vi "piano UI 2.vi"() -> ()   [LabVIEW 2020]
uses:
  midi/midi.lvclass
  midi-file/midi-file.lvclass
  midi-ui/midi-ui.lvclass
  midi/midi.lvclass/midi.ctl
  midi-ui/midi-ui.lvclass/midi-ui.ctl
  <vilib>/addons/_JKI Toolkits/State Machine/_JKI_lib_State_Machine.llb/Select State(s)_err__jki_lib_state_machine.vi
panel:
  in  "Pause":bool
  in  "Stop":bool
  out "Connected?":bool
  in  "Play":bool
  in  "MIDI Out Channel":u32
  in  "Connect MIDI OUT":bool
  in  "Note Length (-1)":dbl=50.0 format="%#_13g"
  in  "Position":enum16{"Top", "Left", "Botom", "Right"}(ring)=enum."Left"
  in  "Load File":bool
  in  "Exit":bool
  out "picture":picture
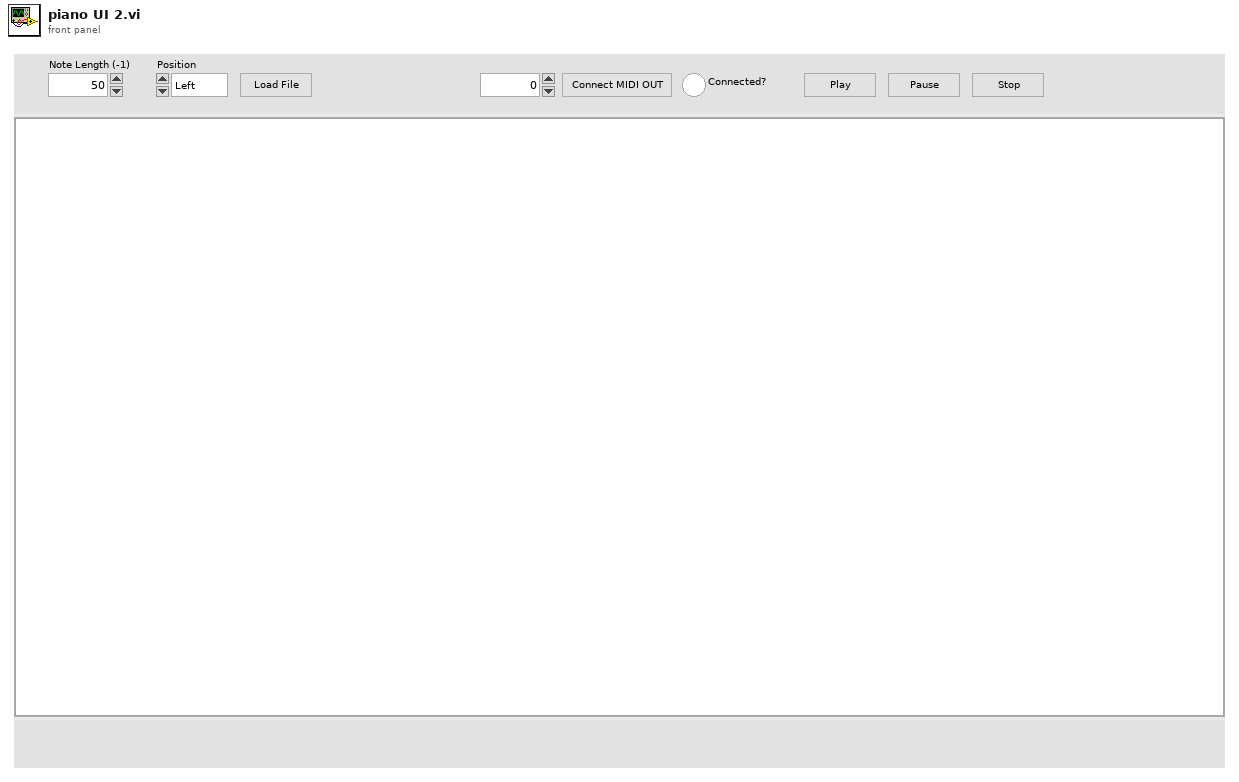
[diagram p1: front panel]
types:
  T1 = enum32{"Invalid", "Standard", "Closed", "Hidden", "Minimized", "Maximized"}
  T2 = enum32{"invalid app kind", "Development System", "Run Time System", "Student Edition", "Embedded LabVIEW", "Evaluation", "Custom"}
  T3 = cluster{"Core":cluster{"Current VI Reference":refnum<vi>, "Close Panel on Exit?":bool}, "MIDI UI obj":refnum<class "midi-ui.lvclass">, "file events":cluster{"Time Delay":u32, "MIDI Messages":u16, "Note Value":enum8{"C-2", "C#-2", "D-2", "D#-2", "E-2", "F-2", "F#-2", "G-2", "G#-2", "A-2", "A#-2", "B-2", "C-1", "C#-1", "D-1", "D#-1", "E-1", "F-1", "F#-1", "G-1", "G#-1", "A-1", "A#-1", "B-1", "C0", "C#0", "D0", "D#0", "E0", "F0", "F#0", "G0", "G#0", "A0", "A#0", "B0", "C1", "C#1", "D1", "D#1", "E1", "F1", "F#1", "G1", "G#1", "A1", "A#1", "B1", "C2", "C#2", "D2", "D#2", "E2", "F2", "F#2", "G2", "G#2", "A2", "A#2", "B2", "C3", "C#3", "D3", "D#3", "E3", "F3", "F#3", "G3", "G#3", "A3", "A#3", "B3", "C4", "C#4", "D4", "D#4", "E4", "F4", "F#4", "G4", "G#4", "A4", "A#4", "B4", "C5", "C#5", "D5", "D#5", "E5", "F5", "F#5", "G5", "G#5", "A5", "A#5", "B5", "C6", "C#6", "D6", "D#6", "E6", "F6", "F#6", "G6", "G#6", "A6", "A#6", "B6", "C7", "C#7", "D7", "D#7", "E7", "F7", "F#7", "G7", "G#7", "A7", "A#7", "B7", "C8", "C#8", "D8", "D#8", "E8", "F8", "F#8", "G"}, "Volume":u8, "uid":i32}[], "file meta events":cluster{"Delta Tiime":u32, "MIDI Meta Events":u16, "String Data":string, "Numeric Data":i32[]}[], "MIDI FILE obj":refnum<class "midi-file.lvclass">, "midi obj":refnum<class "midi.lvclass">, "midi connected?":bool}
  T4 = cluster{"Time Delay":u32, "MIDI Messages":u16, "Note Value":enum8{"C-2", "C#-2", "D-2", "D#-2", "E-2", "F-2", "F#-2", "G-2", "G#-2", "A-2", "A#-2", "B-2", "C-1", "C#-1", "D-1", "D#-1", "E-1", "F-1", "F#-1", "G-1", "G#-1", "A-1", "A#-1", "B-1", "C0", "C#0", "D0", "D#0", "E0", "F0", "F#0", "G0", "G#0", "A0", "A#0", "B0", "C1", "C#1", "D1", "D#1", "E1", "F1", "F#1", "G1", "G#1", "A1", "A#1", "B1", "C2", "C#2", "D2", "D#2", "E2", "F2", "F#2", "G2", "G#2", "A2", "A#2", "B2", "C3", "C#3", "D3", "D#3", "E3", "F3", "F#3", "G3", "G#3", "A3", "A#3", "B3", "C4", "C#4", "D4", "D#4", "E4", "F4", "F#4", "G4", "G#4", "A4", "A#4", "B4", "C5", "C#5", "D5", "D#5", "E5", "F5", "F#5", "G5", "G#5", "A5", "A#5", "B5", "C6", "C#6", "D6", "D#6", "E6", "F6", "F#6", "G6", "G#6", "A6", "A#6", "B6", "C7", "C#7", "D7", "D#7", "E7", "F7", "F#7", "G7", "G#7", "A7", "A#7", "B7", "C8", "C#8", "D8", "D#8", "E8", "F8", "F#8", "G"}, "Volume":u8, "uid":i32}[]
  T5 = cluster{"Delta Tiime":u32, "MIDI Meta Events":u16, "String Data":string, "Numeric Data":i32[]}[]
  T6 = cluster{"Current VI Reference":refnum<vi>, "Close Panel on Exit?":bool}
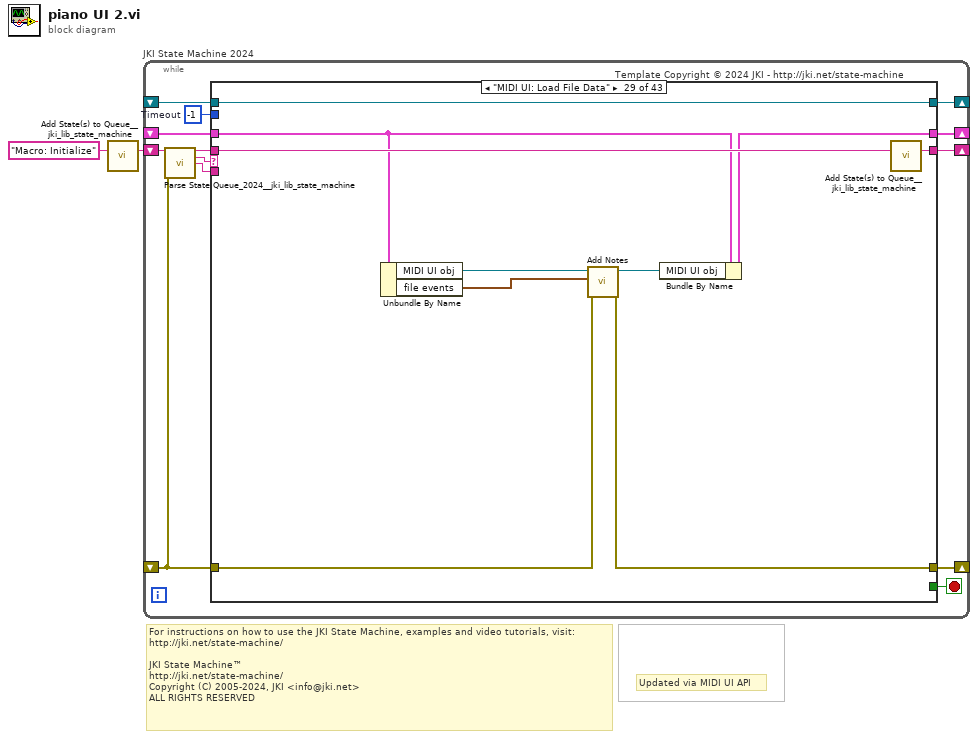
[diagram p0: block diagram]
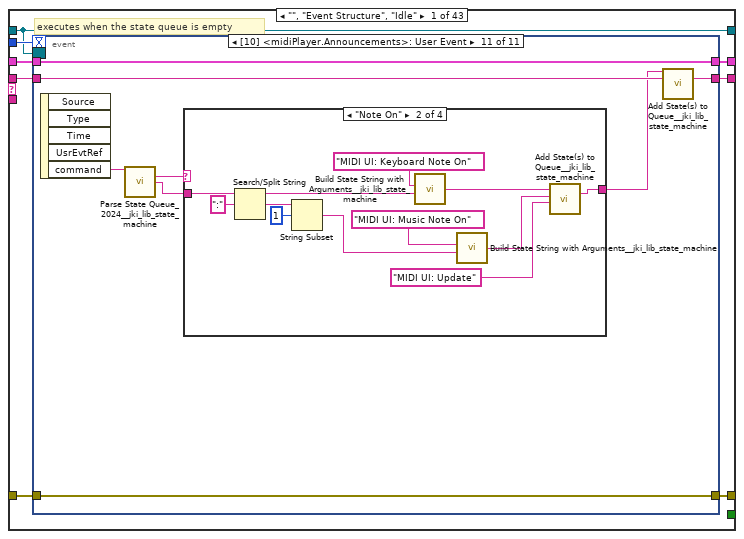
[diagram p2: hidden frame]
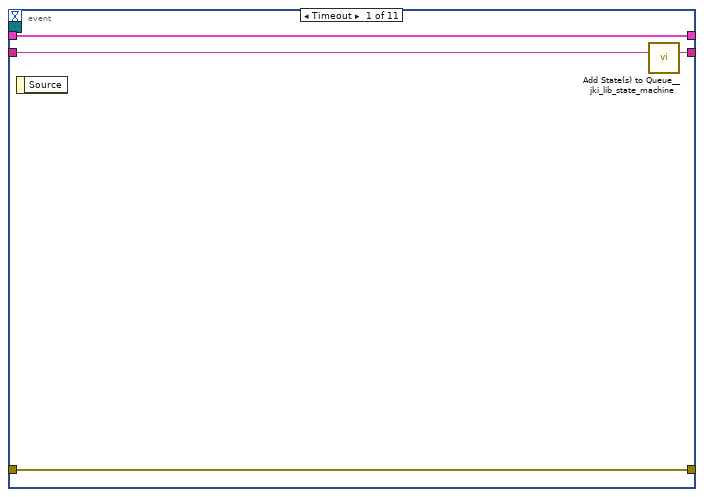
[diagram p3: hidden frame]
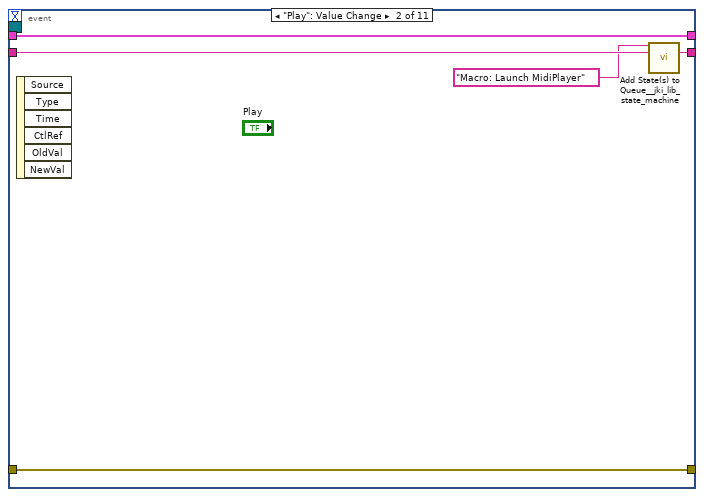
[diagram p4: hidden frame]
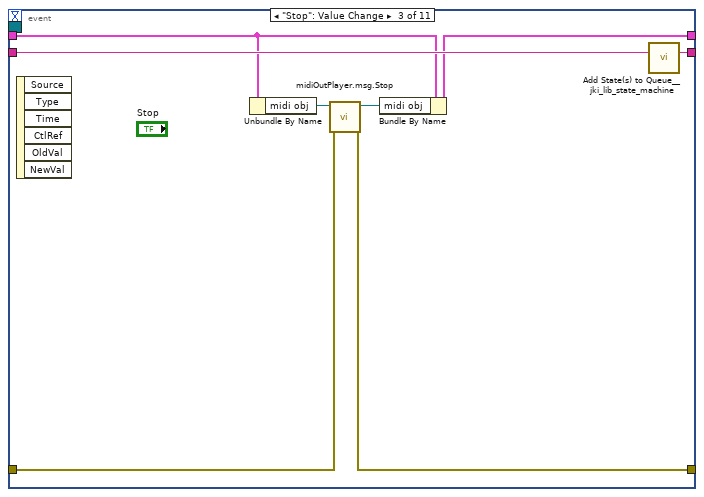
[diagram p5: hidden frame]
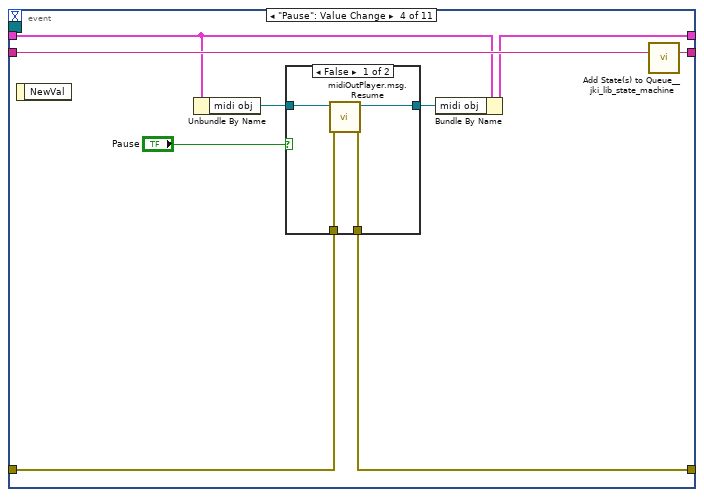
[diagram p6: hidden frame]
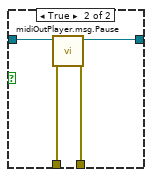
[diagram p7: hidden frame]
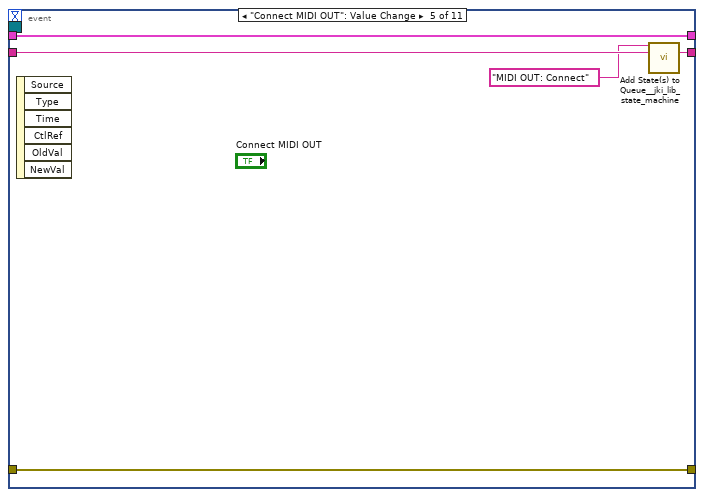
[diagram p8: hidden frame]
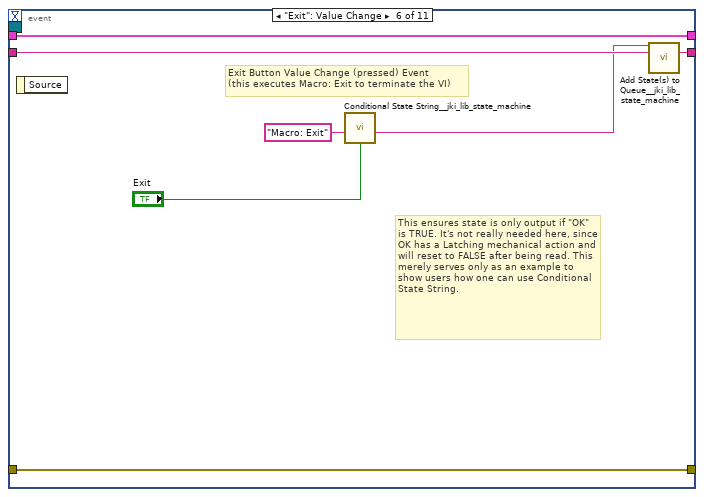
[diagram p9: hidden frame]
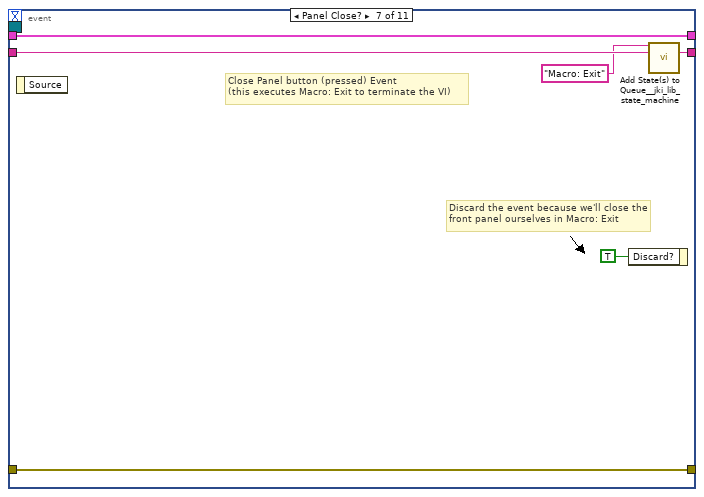
[diagram p10: hidden frame]
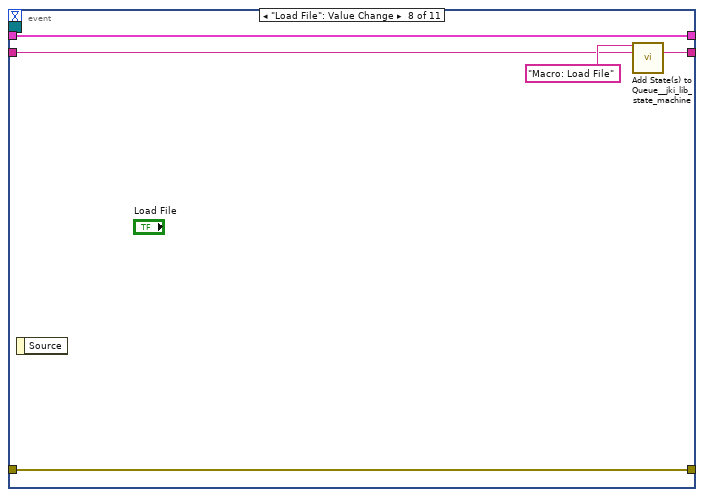
[diagram p11: hidden frame]
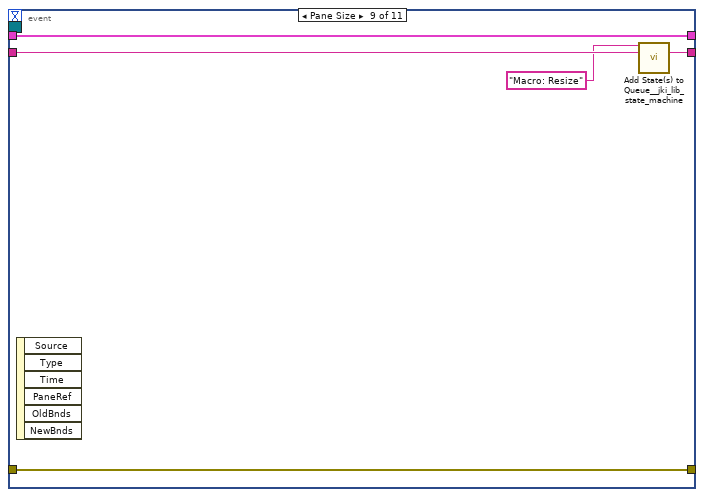
[diagram p12: hidden frame]
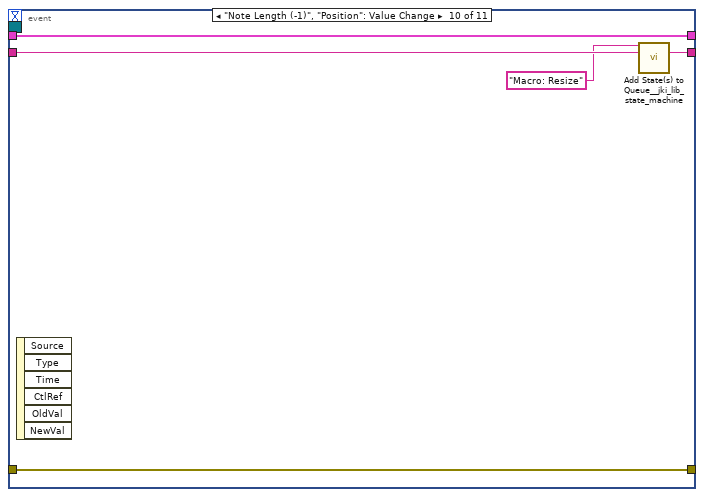
[diagram p13: hidden frame]
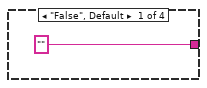
[diagram p14: hidden frame]
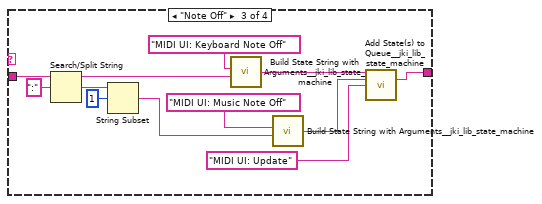
[diagram p15: hidden frame]
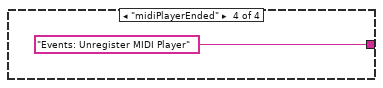
[diagram p16: hidden frame]
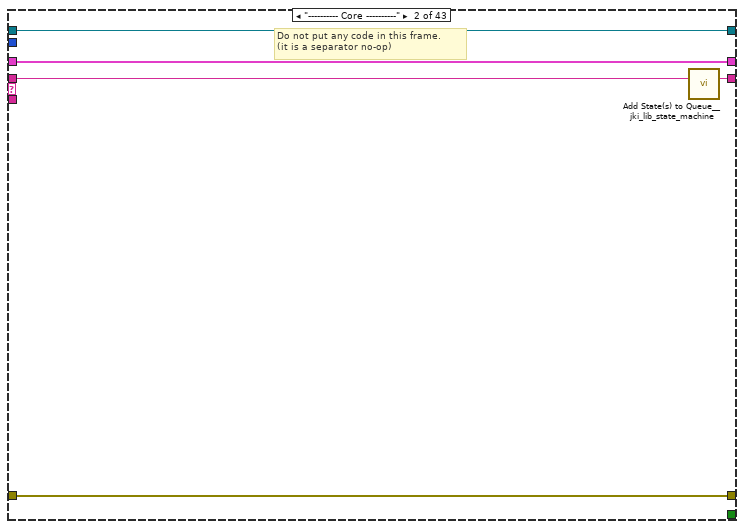
[diagram p17: hidden frame]
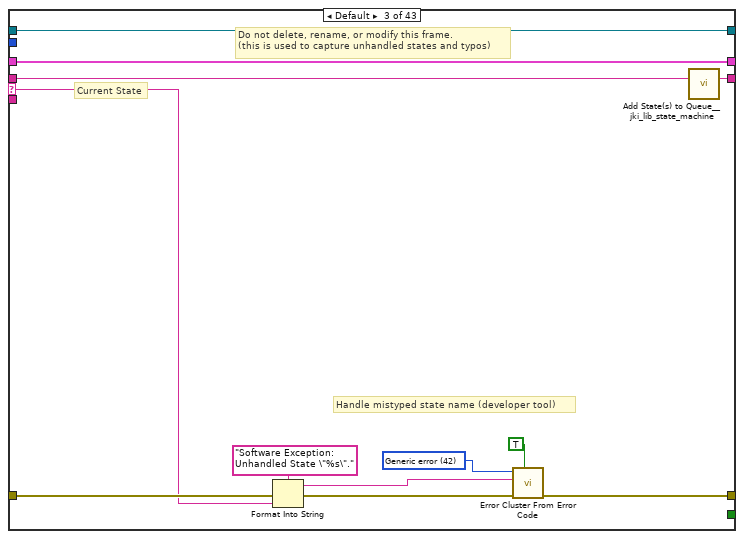
[diagram p18: hidden frame]
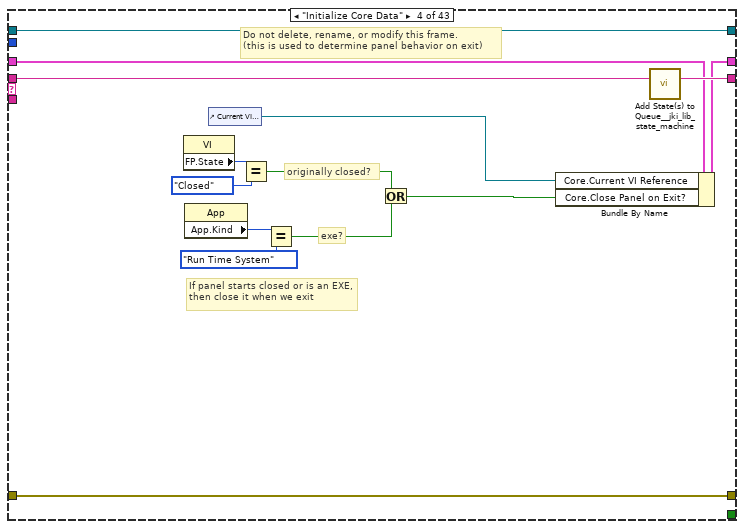
[diagram p19: hidden frame]
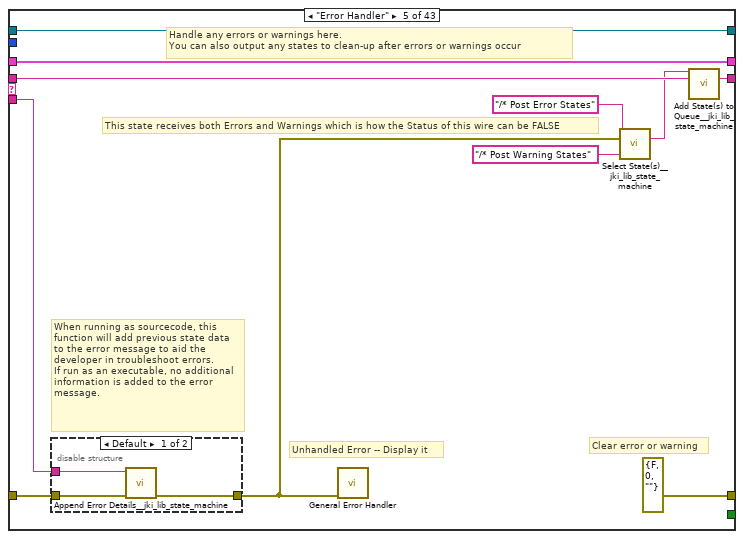
[diagram p20: hidden frame]
diagram:
  # "Updated via MIDI UI API"
  # "For instructions on how to use the JKI State Machine, examples and video tutorials, visit:\nhttp://jki.net/state-machine/\n\nJKI State Machine™\nhttp://jki.net/state-machine/\nCopyright (C) 2005-2024, JKI <info@jki.net>\nALL RIGHTS RESERVED"
  n1 = call <vilib>:"Add State(s) to Queue__jki_lib_state_machine.vi"("State(s) in (\"\")"="Macro: Initialize") -> ("States Out"=w2:string)  [unwired: 14 in]
  n2 = while "JKI State Machine 2024" {
    shift-right: [w10] -> _
    shift-left: _ -> [w9]
    shift-right: [w13] -> _
    shift-left: _ -> [w7]
    shift-right: [w12] -> _
    shift-left: w2 -> [w14]
    shift-right: [w4] -> _
    shift-left: _ -> [w3]
    stop <- w11 stop-if-true
    w8 = -1  # Timeout
    # "Template Copyright © 2024 JKI - http://jki.net/state-machine"
    n3 = call <vilib>:"Parse State Queue_2024__jki_lib_state_machine.vi"("State Queue"=w14, "Error In (no error)"=w7) -> ("Remaining States"=w15:string, "Current State"=w5:string, "Arguments"=w6:string)  [unwired: 11 in]
    n4 = case shown="\"MIDI UI: Load File Data\"" w5 {
      selector: w5 -> [_ _ w131 _ _ _ _ _ _ _ _ _ _ _ _ _ _ _ _ _ _ _ _ _ _ _ _ _ _ _ _ _ _ _ _ _ _ _ _ _ _ _ _]
      tunnel: w15 -> [w23 w129 w135 w155 w166 w176 w181 w198 w205 w210 w217 w226 w234 w240 w245 w251 w256 w263 w275 w345 w351 w357 w363 w369 w382 w387 w394 w408 w418 w430 w440 w450 w460 w470 w473 w482 w493 w500 w505 w516 w526 w536 w545]
      tunnel: w6 -> [_ _ _ _ w161 _ _ _ _ _ _ _ _ _ _ _ _ w258 w269 _ _ _ _ _ _ _ _ _ _ _ w433 w443 w453 w463 _ _ _ _ _ _ _ _ _]
      tunnel: w9 -> [w21 w126 w133 w148 w163 w174 w178 _ w200 w207 w215 w221 w232 w238 w242 w249 w254 w261 w271 w342 w348 w354 w360 w366 w380 w384 w391 w404 w411 w422 w438 w448 w458 w468 w475 w480 w489 w499 w504 w511 w522 w530 w541]
      tunnel: [w20 w127 w137 w152 errorcluster {"status"=FALSE, "code"=0, "source"=""} ("error out") w173 w179 w190 w201 w208 w214 w224 w231 w235 w243 w248 w253 w259 w272 w343 w349 w355 w361 w367 w377 w385 w388 w401 w410 w424 w431 w441 w451 w461 w472 w478 w486 w496 w503 w508 w520 w531 w539] -> w13
      tunnel: w7 -> [w17 w127 w136 w152 w162 w173 w179 w193 w202 w208 w213 w223 w230 w236 w243 w248 w253 w260 w273 w343 w349 w355 w361 w367 w377 w385 w388 w396 w414 w425 w432 w442 w452 w462 w472 w481 w487 w497 w503 w514 w521 w532 w540]
      tunnel: [w22 w128 w134 w154 w165 w175 w180 w197 w204 w209 w216 w225 w233 w239 w244 w250 w255 w262 w274 w344 w350 w356 w362 w368 w381 w386 w393 w407 w417 w429 w439 w449 w459 w469 w474 w483 w494 w501 w506 w517 w527 w537 w546] -> w12
      tunnel: [_ _ _ _ _ TRUE _ _ _ _ _ _ _ _ _ _ _ _ _ _ _ _ _ _ _ _ _ _ _ _ _ _ _ _ _ _ _ _ _ _ _ _ _] -> w11
      tunnel: [w19 w126 w133 w153 w163 w174 w178 w196 w200 w207 w215 w221 w232 w238 w242 w249 w254 w261 w271 w342 w348 w354 w360 w366 w380 w384 w391 w403 w412 w421 w437 w447 w457 w467 w475 w479 w492 w499 w504 w512 w525 w529 w538] -> w10
      tunnel: w8 -> [w18 _ _ _ _ _ _ _ _ _ _ _ _ _ _ _ _ _ _ _ _ _ _ _ _ _ _ _ _ _ _ _ _ _ _ _ _ _ _ _ _ _ _]
      tunnel: [w16 w125 w130 w142 w156 w171 w177 w184 w199 w206 w211 w219 w227 w237 w241 w247 w252 w257 w268 w341 w347 w352 w358 w364 w374 w383 w392 w395 w409 w419 w436 w446 w456 w466 w471 w476 w484 w495 w502 w509 w519 w535 w544] -> w4
      tunnel: w3 -> [w16 w125 w130 w142 w156 w171 w177 w184 w199 w206 w212 w218 w229 w237 w241 w247 w252 w257 w268 w341 w347 w352 w358 w364 w374 w383 w392 w395 w409 w419 w436 w446 w456 w466 w471 w476 w484 w495 w502 w509 w519 w535 w544]
      frame "", "Event Structure", "Idle" {
        # "executes when the state queue is empty"
        n5 = event shown="[10] <midiPlayer.Announcements>: User Event" {
          selector: w16 -> [_ _ _ _ _ _ _ _ _ _ _]
          dyn-events: _ -> [_ _ _ _ _ _ _ _ _ _ _]
          timeout: w18 -> [_ _ _ _ _ _ _ _ _ _ _]
          tunnel: w23 -> [w27 w32 w40 w49 w62 w69 w75 w79 w83 w88 w96]
          tunnel: [w26 w31 w39 w48 w61 w68 w74 w78 w84 w89 w97] -> w22
          tunnel: w21 -> [w24 w29 w37 w46 w59 w66 w72 w77 w85 w90 w91]
          tunnel: [w25 w30 w33 w42 w60 w67 w73 w76 w82 w87 w98] -> w20
          tunnel: w17 -> [w25 w30 w34 w43 w60 w67 w73 w76 w82 w87 w98]
          tunnel: [w24 w29 w36 w45 w59 w66 w72 w77 w85 w90 w91] -> w19
          event Timeout {
            n6 = event-data() -> ()  [unwired: 1 in, 1 out]
            n7 = call <vilib>:"Add State(s) to Queue__jki_lib_state_machine.vi"("State(s) in (\"\")"=w27) -> ("States Out"=w26:string)  [unwired: 14 in]
          }
          event "Play": Value Change {
            n8 = event-data() -> ()  [unwired: 1 in, 6 out]
            n9 = call <vilib>:"Add State(s) to Queue__jki_lib_state_machine.vi"("State(s) in Front (\"\")"="Macro: Launch MidiPlayer" ("State(s) in Front (\"\")"), "State(s) in (\"\")"=w32) -> ("States Out"=w31:string)  [unwired: 13 in]
          }
          event "Stop": Value Change {
            n10 = event-data() -> ()  [unwired: 1 in, 6 out]
            n11 = Unbundle By Name(w37) -> ("midi obj"=w38:refnum<class "midi.lvclass">)
            n12 = call "midiOutPlayer.msg.Stop.vi"("error in (no error)"=w34, "midi in"=w38) -> ("error out"=w33:errorcluster, "midi out"=w35:refnum<class "midi.lvclass">)  [unwired: 8 in]
            n13 = Bundle By Name(cluster=w37, "midi obj"=w35) -> (w36:T3)
            n14 = call <vilib>:"Add State(s) to Queue__jki_lib_state_machine.vi"("State(s) in (\"\")"=w40) -> ("States Out"=w39:string)  [unwired: 14 in]
          }
          event "Pause": Value Change {
            n15 = event-data() -> ()  [unwired: 1 in, 1 out]
            n16 = Unbundle By Name(w46) -> ("midi obj"=w47:refnum<class "midi.lvclass">)
            n17 = case shown="False" "Pause" {
              tunnel: w47 -> [w53 w57]
              tunnel: [w51 w56] -> w44
              tunnel: w43 -> [w52 w55]
              tunnel: [w50 w54] -> w42
              frame False {
                n18 = call "midiOutPlayer.msg.Resume.vi"("error in (no error)"=w52, "midi in"=w53) -> ("error out"=w50:errorcluster, "midi out"=w51:refnum<class "midi.lvclass">)  [unwired: 8 in]
              }
              frame True {
                n19 = call "midiOutPlayer.msg.Pause.vi"("error in (no error)"=w55, "midi in"=w57) -> ("error out"=w54:errorcluster, "midi out"=w56:refnum<class "midi.lvclass">)  [unwired: 8 in]
              }
            }
            n20 = Bundle By Name(cluster=w46, "midi obj"=w44) -> (w45:T3)
            n21 = call <vilib>:"Add State(s) to Queue__jki_lib_state_machine.vi"("State(s) in (\"\")"=w49) -> ("States Out"=w48:string)  [unwired: 14 in]
          }
          event "Connect MIDI OUT": Value Change {
            n22 = event-data() -> ()  [unwired: 1 in, 6 out]
            n23 = call <vilib>:"Add State(s) to Queue__jki_lib_state_machine.vi"("State(s) in Front (\"\")"="MIDI OUT: Connect" ("State(s) in Front (\"\")"), "State(s) in (\"\")"=w62) -> ("States Out"=w61:string)  [unwired: 13 in]
          }
          event "Exit": Value Change {
            # "This ensures state is only output if \"OK\" is TRUE. It's not really needed here, since OK has a Latching mechanical action and will reset to FALSE after being read. This merely serves only as an example to show users how one can use Conditional State String."
            # "Exit Button Value Change (pressed) Event\n(this executes Macro: Exit to terminate the VI)"
            n24 = event-data() -> ()  [unwired: 1 in, 1 out]
            n25 = call <vilib>:"Conditional State String__jki_lib_state_machine.vi"("Do State(s)?"="Exit", "State"="Macro: Exit") -> ("State Out"=w63:string)  [unwired: 7 in]
            n26 = call <vilib>:"Add State(s) to Queue__jki_lib_state_machine.vi"("State(s) in Front (\"\")"=w63, "State(s) in (\"\")"=w69) -> ("States Out"=w68:string)  [unwired: 13 in]
          }
          event Panel Close? {
            # "Discard the event because we'll close the front panel ourselves in Macro: Exit"
            # "Close Panel button (pressed) Event\n(this executes Macro: Exit to terminate the VI)"
            n27 = event-data() -> ()  [unwired: 1 in, 1 out]
            n28 = event-data("Discard?"=TRUE) -> ()  [unwired: 1 in, 1 out]
            n29 = call <vilib>:"Add State(s) to Queue__jki_lib_state_machine.vi"("State(s) in Front (\"\")"="Macro: Exit", "State(s) in (\"\")"=w75) -> ("States Out"=w74:string)  [unwired: 13 in]
          }
          event "Load File": Value Change {
            n30 = event-data() -> ()  [unwired: 1 in, 1 out]
            n31 = call <vilib>:"Add State(s) to Queue__jki_lib_state_machine.vi"("State(s) in Front (\"\")"="Macro: Load File", "State(s) in (\"\")"=w79) -> ("States Out"=w78:string)  [unwired: 13 in]
          }
          event Pane Size {
            n32 = event-data() -> ()  [unwired: 1 in, 6 out]
            n33 = call <vilib>:"Add State(s) to Queue__jki_lib_state_machine.vi"("State(s) in Front (\"\")"="Macro: Resize" ("State(s) in Front (\"\")"), "State(s) in (\"\")"=w83) -> ("States Out"=w84:string)  [unwired: 13 in]
          }
          event "Note Length (-1)", "Position": Value Change {
            n34 = event-data() -> ()  [unwired: 1 in, 6 out]
            n35 = call <vilib>:"Add State(s) to Queue__jki_lib_state_machine.vi"("State(s) in Front (\"\")"="Macro: Resize" ("State(s) in Front (\"\")"), "State(s) in (\"\")"=w88) -> ("States Out"=w89:string)  [unwired: 13 in]
          }
          event User Event {
            n36 = event-data() -> ("command"=w95:string)  [unwired: 1 in, 4 out]
            n37 = call <vilib>:"Parse State Queue_2024__jki_lib_state_machine.vi"("State Queue"=w95) -> ("Current State"=w94:string, "Arguments"=w92:string)  [unwired: 12 in, 1 out]
            n38 = case shown="\"Note On\"" w94 {
              tunnel: ["" ("State(s) in Front (\"\")") w101 w123 "Events: Unregister MIDI Player" ("State(s) in Front (\"\")")] -> w93
              tunnel: w92 -> [_ w100 w118 _]
              frame "False", Default {
              }
              frame "Note On" {
                n39 = Search/Split String(string=w100, search string/char (-)=":") -> (substring before match=w108:string, match + rest of string=w107:string)  [unwired: 1 in, 1 out]
                n40 = String Subset(string=w107, offset (0)=1) -> (substring=w103:string)  [unwired: 1 in]
                n41 = call <vilib>:"Build State String with Arguments__jki_lib_state_machine.vi"("Arguments (\"\")"=w108, "State"="MIDI UI: Keyboard Note On" ("State(s) in Front (\"\")")) -> ("State with Arguments"=w110:string)  [unwired: 4 in]
                n42 = call <vilib>:"Build State String with Arguments__jki_lib_state_machine.vi"("Arguments (\"\")"=w103, "State"="MIDI UI: Music Note On" ("State(s) in Front (\"\")")) -> ("State with Arguments"=w102:string)  [unwired: 4 in]
                n43 = call <vilib>:"Add State(s) to Queue__jki_lib_state_machine.vi"("State(s) in Front (\"\")"=w110, "State(s) in (\"\")"=w102, "State(s) at Back (\"\")"="MIDI UI: Update" ("State(s) in (\"\")")) -> ("States Out"=w101:string)  [unwired: 12 in]
              }
              frame "Note Off" {
                n44 = Search/Split String(string=w118, search string/char (-)=":") -> (substring before match=w119:string, match + rest of string=w117:string)  [unwired: 1 in, 1 out]
                n45 = String Subset(string=w117, offset (0)=1) -> (substring=w113:string)  [unwired: 1 in]
                n46 = call <vilib>:"Build State String with Arguments__jki_lib_state_machine.vi"("Arguments (\"\")"=w119, "State"="MIDI UI: Keyboard Note Off" ("State(s) in Front (\"\")")) -> ("State with Arguments"=w121:string)  [unwired: 4 in]
                n47 = call <vilib>:"Build State String with Arguments__jki_lib_state_machine.vi"("Arguments (\"\")"=w113, "State"="MIDI UI: Music Note Off" ("State(s) in Front (\"\")")) -> ("State with Arguments"=w112:string)  [unwired: 4 in]
                n48 = call <vilib>:"Add State(s) to Queue__jki_lib_state_machine.vi"("State(s) in Front (\"\")"=w121, "State(s) in (\"\")"=w112, "State(s) at Back (\"\")"="MIDI UI: Update" ("State(s) in (\"\")")) -> ("States Out"=w123:string)  [unwired: 12 in]
              }
              frame "midiPlayerEnded" {
              }
            }
            n49 = call <vilib>:"Add State(s) to Queue__jki_lib_state_machine.vi"("State(s) in Front (\"\")"=w93, "State(s) in (\"\")"=w96) -> ("States Out"=w97:string)  [unwired: 13 in]
          }
        }
      }
      frame "---------- Core ----------" {
        # "Do not put any code in this frame.\n(it is a separator no-op)"
        n50 = call <vilib>:"Add State(s) to Queue__jki_lib_state_machine.vi"("State(s) in (\"\")"=w129) -> ("States Out"=w128:string)  [unwired: 14 in]
      }
      frame Default {
        w140 = 42 items=["No error", "Argument error", "Memory is full", "Out of zone", "End of file", "File already open", "Generic file I/O error", "File not found", "File permission error", "Disk is full", "Duplicate path", "Too many files open", "System feature not enabled", "Resource file not found", "Cannot add resource", "Resource not found", "Image not found", "Image memory error", "Pen does not exist", "Config type invalid", "Config token not found", "Config parse error", "Config memory error", "Bad external code format", "Bad external code offset", "External code not present", "Null window", "Destroy window error", "Null menu", "Print aborted", "Bad print record", "Print driver error", "Windows error during printing", "Memory error during printing", "Print dialog error", "Generic print error", "Invalid device refnum", "Device not found", "Device parameter error", "Device unit error", "Cannot open device", "Device call aborted", "Generic error", "Cancelled by user", "Object ID too low", "Object ID too high", "Object not in heap", "Unknown heap", "Unknown object (invalid DefProc)", "Unknown object (DefProc not in table)", "Message out of range", "Invalid (null) method", "Unknown message", "Manager call not supported", "Bad address", "Network operation in progress", "Network operation timed out", "Connection is busy", "Network attribute not supported", "Network error", "Address in use", "System out of memory", "Connection aborted", "Connection refused", "Not connected", "Already connected", "Connection closed", "Initialization error (interapplication manager)", "Bad occurrence", "Wait on unbound occurrence handler", "Occurrence queue overflow", "Datalog type conflict", "Unused", "Unrecognized type (interapplication manager)", "Memory corrupt", "Failed to make temporary DLL", "Old CIN version", "Drag socket not found", "Failed to load drop-object", "Failed to register OLE object", "Failed to release OLE object", "Format specifier type mismatch", "Unknown format specifier", "Too few format specifiers", "Too many format specifiers", "Scan failed", "Newer CIN version", "Error converting to variant", "Runtime menu error", "Password tampered", "Variant attribute not found", "Incompatible variant data type", "Event data is not available", "Event Store is not present", "Occurrence is not found", "Event Queue is not created", "Event info is not available", "Refnum passed is NULL", "Error retrieving Class GUID", "Error retrieving CoClass GUID", "Error retrieving TypeLib GUID.", "Bad built application magic bytes.", "Specific driver is different from the specific driver associated with the Logical Name.", "There is no session opened to the class driver.", "Max Error", "MAX - Error with config objects", "MAX - Error loading configuration", "MAX - Group not supported"]
        # "Current State"
        # "Do not delete, rename, or modify this frame.\n(this is used to capture unhandled states and typos)"
        # "Handle mistyped state name (developer tool)"
        n51 = Format Into String(format string="Software Exception: Unhandled State \"%s\"." ("message"), error in=w136, w131) -> (resulting string=w139:string, error out=w138:errorcluster)  [unwired: 1 in]
        n52 = call <vilib>:"Error Cluster From Error Code.vi"("show call chain? (False)"=TRUE, "error in (no error)"=w138, "error message (\"\")"=w139, "error code (0)"=w140) -> ("error out"=w137:errorcluster)  [unwired: 5 in]
        n53 = call <vilib>:"Add State(s) to Queue__jki_lib_state_machine.vi"("State(s) in (\"\")"=w135) -> ("States Out"=w134:string)  [unwired: 14 in]
      }
      frame "Initialize Core Data" {
        # "Do not delete, rename, or modify this frame.\n(this is used to determine panel behavior on exit)"
        # "originally closed?"
        # "exe?"
        # "If panel starts closed or is an EXE, then close it when we exit"
        n54 = property class="VI"() -> ("FP.State"=w145:T1)  [unwired: 2 in, 2 out]
        n55 = property class="App"() -> ("App.Kind"=w151:T2)  [unwired: 2 in, 2 out]
        n56 = control-ref of="Current VI Reference"() -> (w146:refnum<vi>)
        n57 = Equal?(x=w145, y=T1."Closed" ("Front Panel Window:State")) -> (x = y?=w143:bool)
        n58 = Equal?(x=w151, y=T2."Run Time System" ("Application:Kind")) -> (x = y?=w149:bool)
        n59 = Or(x=w143, y=w149) -> (x .or. y?=w147:bool)
        n60 = Bundle By Name(cluster=w148, "Core.Current VI Reference"=w146, "Core.Close Panel on Exit?"=w147) -> (w153:T3)
        n61 = call <vilib>:"Add State(s) to Queue__jki_lib_state_machine.vi"("State(s) in (\"\")"=w155) -> ("States Out"=w154:string)  [unwired: 14 in]
      }
      frame "Error Handler" {
        # "When running as sourcecode, this function will add previous state data to the error message to aid the developer in troubleshoot errors.\nIf run as an executable, no additional information is added to the error message."
        # "This state receives both Errors and Warnings which is how the Status of this wire can be FALSE"
        # "Unhandled Error -- Display it"
        # "Handle any errors or warnings here.\nYou can also output any states to clean-up after errors or warnings occur"
        # "Clear error or warning"
        n62 = disable-structure shown="Default" {
          disable-tunnel: w162 -> [w169 w170]
          disable-tunnel: w161 -> [w168 _]
          disable-tunnel: [w167 w170] -> w160
          frame condition #0 (active) {
            n63 = call <vilib>:"Append Error Details__jki_lib_state_machine.vi"("error in (no error)"=w169, "Previous State and Argument(s)"=w168) -> ("error out"=w167:errorcluster)  [unwired: 9 in]
          }
          frame condition #1 {
          }
        }
        n64 = call <vilib>:"General Error Handler.vi"("error in (no error)"=w160) -> ()  [unwired: 10 in, 5 out]
        n65 = call-poly <vilib>:"Select State(s)__jki_lib_state_machine.vi"("State(s) if True (\"\")"="/* Post Error States", "Select"=w160, "State(s) if False (\"\")"="/* Post Warning States") -> ("States Out"=w158:string)  [unwired: 12 in]
        n66 = call <vilib>:"Add State(s) to Queue__jki_lib_state_machine.vi"("State(s) in Front (\"\")"=w158, "State(s) in (\"\")"=w166) -> ("States Out"=w165:string)  [unwired: 13 in]
      }
      frame "Exit" {
        # "Do not put any code in this frame.\n(No errors that occur here will be handled.)"
        n67 = call <vilib>:"Add State(s) to Queue__jki_lib_state_machine.vi"("State(s) in (\"\")"=w176) -> ("States Out"=w175:string)  [unwired: 14 in]
      }
      frame "---------- Data ----------" {
        # "Do not put any code in this frame.\n(It is a separator no-op. You can make a copy of this frame to create a new Data frame)"
        n68 = call <vilib>:"Add State(s) to Queue__jki_lib_state_machine.vi"("State(s) in (\"\")"=w181) -> ("States Out"=w180:string)  [unwired: 14 in]
      }
      frame "Data: Initialize" {
        w182 = T4 []  # file events
        w183 = FALSE  # midi connected?
        w185 = refnum<class "midi.lvclass"> refnum  # midi obj
        w188 = refnum<class "midi-file.lvclass"> refnum  # MIDI FILE obj
        w189 = T5 []  # file meta events
        w191 = refnum<class "midi-ui.lvclass"> refnum  # MIDI UI obj
        w195 = T6 {"Current VI Reference"=refnum, "Close Panel on Exit?"=FALSE}  # Core
        # "Data names and types of shift register data are defined by this bundle."
        # "Initialize the shift-register data, here.\n(data names are defined by what you wire into the bundle function)"
        n69 = control-ref of="picture"() -> (w194:refnum<vi>)
        n70 = call "create.vi"("Picture Control"=w194, "error in (no error)"=w193) -> ("error out"=w186:errorcluster, "midi-ui out"=w187:refnum<class "midi-ui.lvclass">)  [unwired: 8 in]
        n71 = Variant To Data(error in=w186, type=w191, Variant=w187) -> (data=w192:refnum<class "midi-ui.lvclass">, error out=w190:errorcluster)
        n72 = Bundle("Core"=w195, "MIDI UI obj"=w192, "file events"=w182, "file meta events"=w189, "MIDI FILE obj"=w188, "midi obj"=w185, "midi connected?"=w183) -> (w196:T3)  [unwired: 1 in]
        n73 = call <vilib>:"Add State(s) to Queue__jki_lib_state_machine.vi"("State(s) in (\"\")"=w198) -> ("States Out"=w197:string)  [unwired: 14 in]
      }
      frame "Data: Cleanup" {
        # "Cleanup any data and references, here.\n(this is called automatically, by the Macro: Exit)"
        n74 = Unbundle By Name(w200) -> ("Core.Current VI Reference"=w203:refnum<vi>)
        n75 = Close Reference(reference=w203, error in (no error)=w202) -> (error out=w201:errorcluster)
        n76 = call <vilib>:"Add State(s) to Queue__jki_lib_state_machine.vi"("State(s) in (\"\")"=w205) -> ("States Out"=w204:string)  [unwired: 14 in]
      }
      frame "---------- Events ----------" {
        # "Do not put any code in this frame.\n(It is a separator no-op. You can make a copy of this frame to create a new UI frame)"
        n77 = call <vilib>:"Add State(s) to Queue__jki_lib_state_machine.vi"("State(s) in (\"\")"=w210) -> ("States Out"=w209:string)  [unwired: 14 in]
      }
      frame "Events: Register" {
        # "Do not put any code in this frame.\n(It is a separator no-op. You can make a copy of this frame to create a new UI frame)"
        n78 = register-events(reference=w212, error in=w213) -> (reference out=w211:refnum<event-registration>, error out=w214:errorcluster)  [unwired: 2 in]
        n79 = call <vilib>:"Add State(s) to Queue__jki_lib_state_machine.vi"("State(s) in (\"\")"=w217) -> ("States Out"=w216:string)  [unwired: 14 in]
      }
      frame "Events: Register MIDI Player" {
        # "Do not put any code in this frame.\n(It is a separator no-op. You can make a copy of this frame to create a new UI frame)"
        n80 = Unbundle By Name(w221) -> ("midi obj"=w220:refnum<class "midi.lvclass">)
        n81 = call "midiPlayer.announcements.get.vi"("midi"=w220) -> ("midiPlayer.Announcements"=w222:refnum<user-event>)  [unwired: 10 in]
        n82 = register-events(reference=w218, error in=w223, w222) -> (reference out=w219:refnum<event-registration>, error out=w224:errorcluster)  [unwired: 1 in]
        n83 = call <vilib>:"Add State(s) to Queue__jki_lib_state_machine.vi"("State(s) in (\"\")"=w226) -> ("States Out"=w225:string)  [unwired: 14 in]
      }
      frame "Events: Unregister MIDI Player" {
        # "Do not put any code in this frame.\n(It is a separator no-op. You can make a copy of this frame to create a new UI frame)"
        n84 = register-events(reference=w229, error in=w230, refnum<user-event> refnum ("event source")) -> (reference out=w227:refnum<event-registration>, error out=w231:errorcluster)  [unwired: 1 in]
        n85 = call <vilib>:"Add State(s) to Queue__jki_lib_state_machine.vi"("State(s) in (\"\")"=w234) -> ("States Out"=w233:string)  [unwired: 14 in]
      }
      frame "Events: Unregister" {
        # "Do not put any code in this frame.\n(It is a separator no-op. You can make a copy of this frame to create a new UI frame)"
        n86 = Unregister For Events(event registration refnum=w237, error in=w236) -> (error out=w235:errorcluster)
        n87 = call <vilib>:"Add State(s) to Queue__jki_lib_state_machine.vi"("State(s) in (\"\")"=w240) -> ("States Out"=w239:string)  [unwired: 14 in]
      }
      frame "---------- UI ----------" {
        # "Do not put any code in this frame.\n(It is a separator no-op. You can make a copy of this frame to create a new UI frame)"
        n88 = call <vilib>:"Add State(s) to Queue__jki_lib_state_machine.vi"("State(s) in (\"\")"=w245) -> ("States Out"=w244:string)  [unwired: 14 in]
      }
      frame "UI: Initialize" {
        # "Initialize the User Interface, here.\n(this is called automatically, by the Macro: Initialize)"
        n89 = local write "Pause"(FALSE ("Pause")) -> ()
        n90 = call <vilib>:"Add State(s) to Queue__jki_lib_state_machine.vi"("State(s) in (\"\")"=w251) -> ("States Out"=w250:string)  [unwired: 14 in]
      }
      frame "UI: Uninitialize" {
        # "Cleanup the User Interface, here.\n(this is called automatically, by the Macro: Exit)"
        n91 = call <vilib>:"Add State(s) to Queue__jki_lib_state_machine.vi"("State(s) in (\"\")"=w256) -> ("States Out"=w255:string)  [unwired: 14 in]
      }
      frame "UI: Cursor Set" {
        # "Argument"
        # "Set and Unset Cursor Busy.\n(Usage: \"UI: Cursor Set >> Busy|Idle\")"
        n92 = case shown="\"Idle\", Default" w258 {
          tunnel: w260 -> [w265 w267]
          tunnel: [w264 w266] -> w259
          frame "Idle", Default {
            n93 = call <vilib>:"Unset Busy.vi"("error in (no error)"=w265) -> ("error out"=w264:errorcluster)  [unwired: 10 in]
          }
          frame "Busy" {
            n94 = call <vilib>:"Set Busy.vi"("error in (no error)"=w267) -> ("error out"=w266:errorcluster)  [unwired: 9 in, 1 out]
          }
        }
        n95 = call <vilib>:"Add State(s) to Queue__jki_lib_state_machine.vi"("State(s) in (\"\")"=w263) -> ("States Out"=w262:string)  [unwired: 14 in]
      }
      frame "UI: Front Panel State" {
        # "Argument"
        # "Set Front Panel Open or Closed\n(Usage: \"UI: Front Panel State >> Open|Close\")"
        n96 = Unbundle By Name(w271) -> ("Core.Current VI Reference"=w270:refnum<vi>)
        n97 = case shown="\"Minimize\", \"Minimized\"" w269 {
          tunnel: w273 -> [w281 w296 w307 w320 w333]
          tunnel: [w283 w297 w309 w322 w335] -> w272
          tunnel: w270 -> [w282 w294 w308 w321 w334]
          frame "Open", "Standard", Default {
            w276 = T1."Standard" ("State")
            n98 = property class="VI"(reference=w282, error in=w281) -> (reference out=w279:refnum<vi>, error out=w280:errorcluster, "FP.State"=w278:T1)
            n99 = Not Equal?(x=w278, y=w276) -> (x != y?=w277:bool)
            n100 = case shown="True" w277 {
              tunnel: [w287 w289] -> w283
              tunnel: w280 -> [w286 w289]
              tunnel: w279 -> [w285 _]
              tunnel: w276 -> [w284 _]
              frame True {
                n101 = invoke class="VI" method="FP.Open"(reference=w285, error in=w286, "Activate"=TRUE, "State"=w284) -> (error out=w287:errorcluster)  [unwired: 1 in, 4 out]
              }
              frame False {
              }
            }
          }
          frame "Close", "Closed" {
            n102 = property class="VI"(reference=w294, error in=w296) -> (reference out=w293:refnum<vi>, error out=w295:errorcluster, "FP.State"=w291:T1)
            n103 = Not Equal?(x=w291, y=T1."Closed" ("Front Panel Window:State")) -> (x != y?=w290:bool)
            n104 = case shown="True" w290 {
              tunnel: [w298 w301] -> w297
              tunnel: w295 -> [w298 w300]
              tunnel: w293 -> [_ w299]
              frame False {
              }
              frame True {
                n105 = invoke class="VI" method="FP.Close"(reference=w299, error in=w300) -> (error out=w301:errorcluster)  [unwired: 1 in, 2 out]
              }
            }
          }
          frame "Hidden", "Hide" {
            w302 = T1."Hidden" ("State")
            n106 = property class="VI"(reference=w308, error in=w307) -> (reference out=w305:refnum<vi>, error out=w306:errorcluster, "FP.State"=w304:T1)
            n107 = Not Equal?(x=w304, y=w302) -> (x != y?=w303:bool)
            n108 = case shown="True" w303 {
              tunnel: [w313 w314] -> w309
              tunnel: w306 -> [w312 w314]
              tunnel: w305 -> [w311 _]
              tunnel: w302 -> [w310 _]
              frame True {
                n109 = invoke class="VI" method="FP.Open"(reference=w311, error in=w312, "State"=w310) -> (error out=w313:errorcluster)  [unwired: 2 in, 4 out]
              }
              frame False {
              }
            }
          }
          frame "Minimize", "Minimized" {
            w315 = T1."Minimized" ("State")
            n110 = property class="VI"(reference=w321, error in=w320) -> (reference out=w318:refnum<vi>, error out=w319:errorcluster, "FP.State"=w317:T1)
            n111 = Not Equal?(x=w317, y=w315) -> (x != y?=w316:bool)
            n112 = case shown="True" w316 {
              tunnel: [w326 w327] -> w322
              tunnel: w319 -> [w325 w327]
              tunnel: w318 -> [w324 _]
              tunnel: w315 -> [w323 _]
              frame True {
                n113 = invoke class="VI" method="FP.Open"(reference=w324, error in=w325, "State"=w323) -> (error out=w326:errorcluster)  [unwired: 2 in, 4 out]
              }
              frame False {
              }
            }
          }
          frame "Maximize", "Maximized" {
            w328 = T1."Maximized" ("State")
            n114 = property class="VI"(reference=w334, error in=w333) -> (reference out=w331:refnum<vi>, error out=w332:errorcluster, "FP.State"=w330:T1)
            n115 = Not Equal?(x=w330, y=w328) -> (x != y?=w329:bool)
            n116 = case shown="True" w329 {
              tunnel: [w339 w340] -> w335
              tunnel: w332 -> [w338 w340]
              tunnel: w331 -> [w337 _]
              tunnel: w328 -> [w336 _]
              frame True {
                n117 = invoke class="VI" method="FP.Open"(reference=w337, error in=w338, "State"=w336) -> (error out=w339:errorcluster)  [unwired: 2 in, 4 out]
              }
              frame False {
              }
            }
          }
        }
        n118 = call <vilib>:"Add State(s) to Queue__jki_lib_state_machine.vi"("State(s) in (\"\")"=w275) -> ("States Out"=w274:string)  [unwired: 14 in]
      }
      frame "---------- Macro ----------" {
        # "Do not put any code in this frame.\n(It is a separator no-op. You can make a copy of this frame to create a new Macro frame)"
        n119 = call <vilib>:"Add State(s) to Queue__jki_lib_state_machine.vi"("State(s) in (\"\")"=w345) -> ("States Out"=w344:string)  [unwired: 14 in]
      }
      frame "Macro: Launch MidiPlayer" {
        n120 = call <vilib>:"Add State(s) to Queue__jki_lib_state_machine.vi"("State(s) in Front (\"\")"="MIDI OUT: Launch Player\nEvents: Register MIDI Player\nMIDI OUT: Play" ("State(s) in Front (\"\")"), "State(s) in (\"\")"=w351) -> ("States Out"=w350:string)  [unwired: 13 in]
      }
      frame "Macro: Initialize" {
        # "Initialization Macro\n(This is called once, when the VI starts)"
        n121 = call <vilib>:"Add State(s) to Queue__jki_lib_state_machine.vi"("State(s) in Front (\"\")"="Data: Initialize\nInitialize Core Data\nEvents: Register\nUI: Initialize\nMIDI UI: Add Keyboard\nMIDI UI: Update\nUI: Front Panel State >> Open", "State(s) in (\"\")"=w357) -> ("States Out"=w356:string)  [unwired: 13 in]
      }
      frame "Macro: Load File" {
        n122 = call <vilib>:"Add State(s) to Queue__jki_lib_state_machine.vi"("State(s) in Front (\"\")"="MIDI FILE: Open File\nUI: Cursor Set >> Busy\nMIDI FILE: Analyse File\nMIDI FILE: Close File\nMIDI UI: Load File Data\nMIDI UI: Update\nUI: Cursor Set >> Idle" ("State(s) in Front (\"\")"), "State(s) in (\"\")"=w363) -> ("States Out"=w362:string)  [unwired: 13 in]
      }
      frame "Macro: Resize" {
        # "Do not put any code in this frame.\n(It is a separator no-op. You can make a copy of this frame to create a new Macro frame)"
        n123 = call <vilib>:"Add State(s) to Queue__jki_lib_state_machine.vi"("State(s) in Front (\"\")"="MIDI UI: Add Keyboard\nMIDI UI: Load File Data\nMIDI UI: Update" ("State(s) in Front (\"\")"), "State(s) in (\"\")"=w369) -> ("States Out"=w368:string)  [unwired: 13 in]
      }
      frame "Macro: Exit" {
        # "Exit Macro\n(This is called once, when the VI exits)"
        n124 = Unbundle By Name(w380) -> ("Core.Close Panel on Exit?"=w375:bool, "midi connected?"=w371:bool)
        n125 = call <vilib>:"Conditional State String__jki_lib_state_machine.vi"("Do State(s)?"=w371, "State"="MIDI OUT: Disconnect") -> ("State Out"=w370:string)  [unwired: 7 in]
        n126 = call <vilib>:"Conditional State String__jki_lib_state_machine.vi"("Do State(s)?"=w375, "State"="UI: Front Panel State >> Close") -> ("State Out"=w373:string)  [unwired: 7 in]
        n127 = call <vilib>:"Add State(s) to Queue__jki_lib_state_machine.vi"("State(s) in Front (\"\")"=w373, "State(s) in (\"\")"=w370, "State(s) at Back (\"\")"="MIDI UI: Clear Screen\nUI: Uninitialize\nData: Cleanup\nEvents: Unregister\nExit") -> ("States Out"=w378:string)  [unwired: 12 in]
        n128 = call <vilib>:"Add State(s) to Queue__jki_lib_state_machine.vi"("State(s) in Front (\"\")"=w378, "State(s) in (\"\")"=w382) -> ("States Out"=w381:string)  [unwired: 13 in]
      }
      frame "---------- MIDI UI ----------" {
        # "Template Separator\n(You can make a copy of, or modify, this frame)"
        n129 = call <vilib>:"Add State(s) to Queue__jki_lib_state_machine.vi"("State(s) in (\"\")"=w387) -> ("States Out"=w386:string)  [unwired: 14 in]
      }
      frame "MIDI UI: Update" {
        n130 = Unbundle By Name(w391) -> ("MIDI UI obj"=w390:refnum<class "midi-ui.lvclass">)
        n131 = call "picture.get2.vi"("midi-ui in"=w390) -> ("image"=→"picture":picture)  [unwired: 10 in]
        n132 = call <vilib>:"Add State(s) to Queue__jki_lib_state_machine.vi"("State(s) in (\"\")"=w394) -> ("States Out"=w393:string)  [unwired: 14 in]
      }
      frame "MIDI UI: Add Keyboard" {
        n133 = Unbundle By Name(w404) -> ("MIDI UI obj"=w399:refnum<class "midi-ui.lvclass">)
        n134 = call "clear picture.vi"("Keep Keyboard? (T)"=FALSE, "error in"=w396, "midi-ui in"=w399) -> ("error out"=w397:errorcluster, "midi-ui out"=w398:refnum<class "midi-ui.lvclass">)  [unwired: 7 in]
        n135 = call "Add Keyboard.vi"("Note Length (-1)"="Note Length (-1)", "error in (no error)"=w397, "Position"="Position", "midi-ui in"=w398) -> ("error out"=w401:errorcluster, "midi-ui out"=w402:refnum<class "midi-ui.lvclass">)  [unwired: 6 in]
        n136 = Bundle By Name(cluster=w404, "MIDI UI obj"=w402) -> (w403:T3)
        n137 = call <vilib>:"Add State(s) to Queue__jki_lib_state_machine.vi"("State(s) in (\"\")"=w408) -> ("States Out"=w407:string)  [unwired: 14 in]
      }
      frame "MIDI UI: Load File Data" {
        n138 = Unbundle By Name(w411) -> ("MIDI UI obj"=w416:refnum<class "midi-ui.lvclass">, "file events"=w415:T4)
        n139 = call "Add Notes.vi"("error in (no error)"=w414, "file events"=w415, "midi-ui in"=w416) -> ("error out"=w410:errorcluster, "midi-ui out"=w413:refnum<class "midi-ui.lvclass">)  [unwired: 7 in]
        n140 = Bundle By Name(cluster=w411, "MIDI UI obj"=w413) -> (w412:T3)
        n141 = call <vilib>:"Add State(s) to Queue__jki_lib_state_machine.vi"("State(s) in (\"\")"=w418) -> ("States Out"=w417:string)  [unwired: 14 in]
      }
      frame "MIDI UI: Clear Screen" {
        n142 = Unbundle By Name(w422) -> ("MIDI UI obj"=w423:refnum<class "midi-ui.lvclass">)
        n143 = call "clear picture.vi"("Keep Keyboard? (T)"=FALSE, "error in"=w425, "midi-ui in"=w423) -> ("error out"=w426:errorcluster, "midi-ui out"=w427:refnum<class "midi-ui.lvclass">)  [unwired: 7 in]
        n144 = call "picture.get.vi"("error in"=w426, "midi-ui in"=w427) -> ("error out"=w424:errorcluster, "midi-ui out"=w420:refnum<class "midi-ui.lvclass">)  [unwired: 8 in]
        n145 = Bundle By Name(cluster=w422, "MIDI UI obj"=w420) -> (w421:T3)
        n146 = call <vilib>:"Add State(s) to Queue__jki_lib_state_machine.vi"("State(s) in (\"\")"=w430) -> ("States Out"=w429:string)  [unwired: 14 in]
      }
      frame "MIDI UI: Keyboard Note On" {
        n147 = Unbundle By Name(w438) -> ("MIDI UI obj"=w435:refnum<class "midi-ui.lvclass">)
        n148 = call "keyboard.NoteOn.vi"("error in (no error)"=w432, "Note On"=w433, "midi-ui in"=w435) -> ("error out"=w431:errorcluster, "midi-ui out"=w434:refnum<class "midi-ui.lvclass">)  [unwired: 7 in]
        n149 = Bundle By Name(cluster=w438, "MIDI UI obj"=w434) -> (w437:T3)
        n150 = call <vilib>:"Add State(s) to Queue__jki_lib_state_machine.vi"("State(s) in (\"\")"=w440) -> ("States Out"=w439:string)  [unwired: 14 in]
      }
      frame "MIDI UI: Music Note On" {
        n151 = Unbundle By Name(w448) -> ("MIDI UI obj"=w445:refnum<class "midi-ui.lvclass">)
        n152 = call "music.NoteOn.vi"("error in (no error)"=w442, "Note On"=w443, "midi-ui in"=w445) -> ("error out"=w441:errorcluster, "midi-ui out"=w444:refnum<class "midi-ui.lvclass">)  [unwired: 7 in]
        n153 = Bundle By Name(cluster=w448, "MIDI UI obj"=w444) -> (w447:T3)
        n154 = call <vilib>:"Add State(s) to Queue__jki_lib_state_machine.vi"("State(s) in (\"\")"=w450) -> ("States Out"=w449:string)  [unwired: 14 in]
      }
      frame "MIDI UI: Keyboard Note Off" {
        n155 = Unbundle By Name(w458) -> ("MIDI UI obj"=w455:refnum<class "midi-ui.lvclass">)
        n156 = call "keyboard.NoteOff.vi"("error in (no error)"=w452, "Note Off"=w453, "midi-ui in"=w455) -> ("error out"=w451:errorcluster, "midi-ui out"=w454:refnum<class "midi-ui.lvclass">)  [unwired: 7 in]
        n157 = Bundle By Name(cluster=w458, "MIDI UI obj"=w454) -> (w457:T3)
        n158 = call <vilib>:"Add State(s) to Queue__jki_lib_state_machine.vi"("State(s) in (\"\")"=w460) -> ("States Out"=w459:string)  [unwired: 14 in]
      }
      frame "MIDI UI: Music Note Off" {
        n159 = Unbundle By Name(w468) -> ("MIDI UI obj"=w465:refnum<class "midi-ui.lvclass">)
        n160 = call "music.NoteOff.vi"("error in (no error)"=w462, "Note Off"=w463, "midi-ui in"=w465) -> ("error out"=w461:errorcluster, "midi-ui out"=w464:refnum<class "midi-ui.lvclass">)  [unwired: 7 in]
        n161 = Bundle By Name(cluster=w468, "MIDI UI obj"=w464) -> (w467:T3)
        n162 = call <vilib>:"Add State(s) to Queue__jki_lib_state_machine.vi"("State(s) in (\"\")"=w470) -> ("States Out"=w469:string)  [unwired: 14 in]
      }
      frame "---------- MIDI FILE ----------" {
        n163 = call <vilib>:"Add State(s) to Queue__jki_lib_state_machine.vi"("State(s) in (\"\")"=w473) -> ("States Out"=w474:string)  [unwired: 14 in]
      }
      frame "MIDI FILE: Open File" {
        n164 = call "file.open.vi"("error in"=w481) -> ("error out"=w478:errorcluster, "midi-file out"=w477:refnum<class "midi-file.lvclass">)  [unwired: 9 in]
        n165 = Bundle By Name(cluster=w480, "MIDI FILE obj"=w477) -> (w479:T3)
        n166 = call <vilib>:"Add State(s) to Queue__jki_lib_state_machine.vi"("State(s) in (\"\")"=w482) -> ("States Out"=w483:string)  [unwired: 14 in]
      }
      frame "MIDI FILE: Analyse File" {
        n167 = Unbundle By Name(w489) -> ("MIDI FILE obj"=w488:refnum<class "midi-file.lvclass">)
        n168 = call "track_chunk.read.vi"("error in"=w487, "midi-file in"=w488) -> ("error out"=w486:errorcluster, "Meta Events"=w490:T5, "MIDI Events"=w491:T4, "midi-file out"=w485:refnum<class "midi-file.lvclass">)  [unwired: 6 in]
        n169 = Bundle By Name(cluster=w489, "MIDI FILE obj"=w485, "file events"=w491, "file meta events"=w490) -> (w492:T3)
        n170 = call <vilib>:"Add State(s) to Queue__jki_lib_state_machine.vi"("State(s) in (\"\")"=w493) -> ("States Out"=w494:string)  [unwired: 14 in]
      }
      frame "MIDI FILE: Close File" {
        n171 = Unbundle By Name(w499) -> ("MIDI FILE obj"=w498:refnum<class "midi-file.lvclass">)
        n172 = call "file.close.vi"("error in"=w497, "midi-file in"=w498) -> ("error out"=w496:errorcluster)  [unwired: 9 in]
        n173 = call <vilib>:"Add State(s) to Queue__jki_lib_state_machine.vi"("State(s) in (\"\")"=w500) -> ("States Out"=w501:string)  [unwired: 14 in]
      }
      frame "---------- MIDI OUT ----------" {
        n174 = call <vilib>:"Add State(s) to Queue__jki_lib_state_machine.vi"("State(s) in (\"\")"=w505) -> ("States Out"=w506:string)  [unwired: 14 in]
      }
      frame "MIDI OUT: Connect" {
        n175 = Unbundle By Name(w511) -> ("midi obj"=w513:refnum<class "midi.lvclass">)
        n176 = call "midiOutOpen.vi"("error in"=w514, "DeviceID"="MIDI Out Channel", "midi in"=w513) -> ("error out"=w508:errorcluster, "midi out"=w510:refnum<class "midi.lvclass">)  [unwired: 7 in]
        n177 = Not(x=w508) -> (.not. x?=w507:bool)
        "Connected?" <- w507
        n178 = Bundle By Name(cluster=w511, "midi obj"=w510, "midi connected?"=w507) -> (w512:T3)
        n179 = call <vilib>:"Add State(s) to Queue__jki_lib_state_machine.vi"("State(s) in (\"\")"=w516) -> ("States Out"=w517:string)  [unwired: 14 in]
      }
      frame "MIDI OUT: Disconnect" {
        w518 = FALSE ("midi connected?")
        n180 = Unbundle By Name(w522) -> ("midi obj"=w523:refnum<class "midi.lvclass">)
        n181 = call "midiOutClose.vi"("error in"=w521, "midi in"=w523) -> ("error out"=w520:errorcluster, "midi out"=w524:refnum<class "midi.lvclass">)  [unwired: 8 in]
        n182 = Bundle By Name(cluster=w522, "midi connected?"=w518, "midi obj"=w524) -> (w525:T3)
        n183 = local write "Connected?"(w518) -> ()
        n184 = call <vilib>:"Add State(s) to Queue__jki_lib_state_machine.vi"("State(s) in (\"\")"=w526) -> ("States Out"=w527:string)  [unwired: 14 in]
      }
      frame "MIDI OUT: Launch Player" {
        n185 = Unbundle By Name(w530) -> ("midi obj"=w534:refnum<class "midi.lvclass">, "file events"=w533:T4)
        n186 = call "midiOutPlayer.Launch.vi"("error in"=w532, "file events"=w533, "midi in"=w534) -> ("error out"=w531:errorcluster, "midi out"=w528:refnum<class "midi.lvclass">)  [unwired: 7 in]
        n187 = Bundle By Name(cluster=w530, "midi obj"=w528) -> (w529:T3)
        n188 = call <vilib>:"Add State(s) to Queue__jki_lib_state_machine.vi"("State(s) in (\"\")"=w536) -> ("States Out"=w537:string)  [unwired: 14 in]
      }
      frame "MIDI OUT: Play" {
        n189 = Unbundle By Name(w541) -> ("midi obj"=w542:refnum<class "midi.lvclass">)
        n190 = call "midiOutPlayer.msg.Play.vi"("error in (no error)"=w540, "midi in"=w542) -> ("error out"=w539:errorcluster, "midi out"=w543:refnum<class "midi.lvclass">)  [unwired: 8 in]
        n191 = Bundle By Name(cluster=w541, "midi obj"=w543) -> (w538:T3)
        n192 = call <vilib>:"Add State(s) to Queue__jki_lib_state_machine.vi"("State(s) in (\"\")"=w545) -> ("States Out"=w546:string)  [unwired: 14 in]
      }
    }
  }
